vi "rs3 Burn_calibration_table.vi"(8 "error in (no error)":errorcluster, 11 "Device in":u64) -> (0 "error out":errorcluster, 1 "error":u64, 3 "Device out":u64)   [LabVIEW 2017, in "libRealSense3.lvlib"]
doc: "STARTS the streaming of a specific sensor, based on the input QUEUE."
uses:
  libRealSense3.lvlib
  realsense2.dll
panel:
  # "RS Burn Calibration Table"
  # "(C) 2019 Intel Corp.,  AGJ"
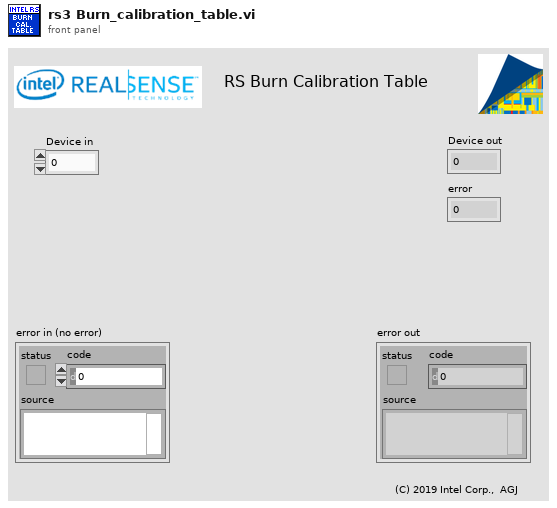
[diagram p1: front panel]
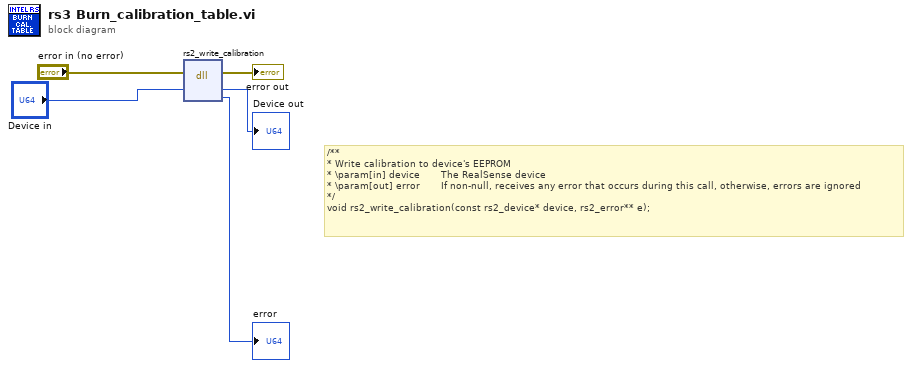
[diagram p0: block diagram]
diagram:
  # "/**\n* Write calibration to device's EEPROM\n* \\param[in] device       The RealSense device\n* \\param[out] error       If non-null, receives any error that occurs during this call, otherwise, errors are ignored\n*/\nvoid rs2_write_calibration(const rs2_device* device, rs2_error** e);"
  n1 = dll-call lib="C:/Users/agrunnet/Documents/libRealSense6/realsense2.dll" fn="rs2_write_calibration"(error in="error in (no error)", "device"="Device in") -> (error out=→"error out":errorcluster, "device"=→"Device out":u64, "error"=→"error":u64)  [unwired: 4 in, 1 out]
